vi "STM Reference FGV.vi"(7 "command":enum16{"Set", "Get"}(ring)=enum."Get", 8 "error in":errorcluster, 9 "STM queue in":refnum<queue>, 10 "TCP listener ID in":refnum<k5>, 11 "TCP connection ID in":refnum<k5>) -> (0 "error ou":errorcluster, 1 "STM queue out":refnum<queue>, 2 "TCP listener ID out":refnum<k5>, 3 "TCP connection ID out":refnum<k5>)   [LabVIEW 2017, in "WinHost.lvlib"]
uses:
  WinHost.lvlib
  Private TypeDefs/STM Queue Element.ctl
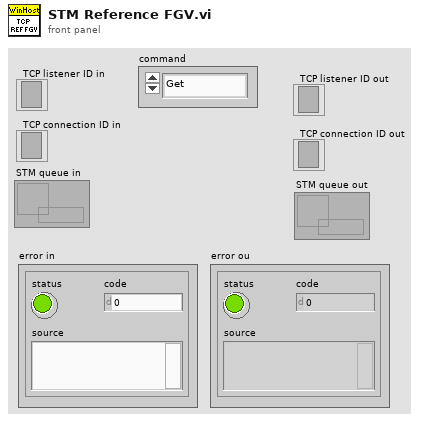
[diagram p1: front panel]
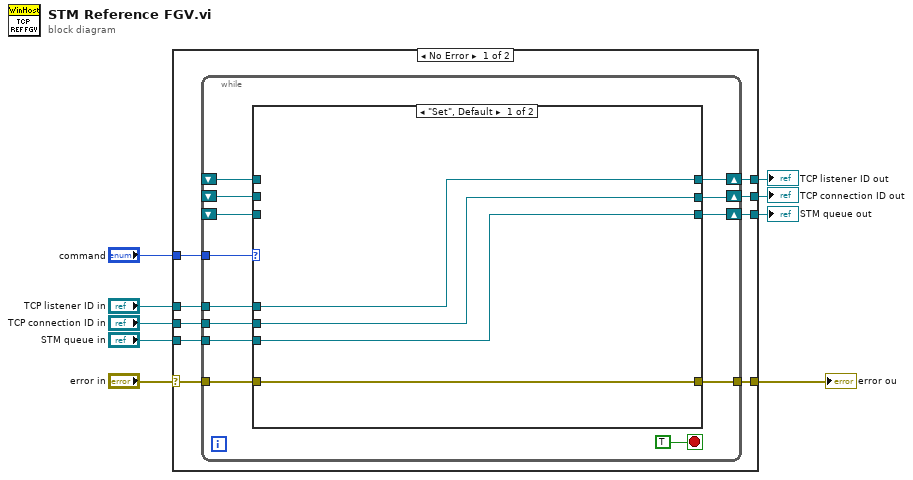
[diagram p0: block diagram]
diagram:
  n1 = case shown="No Error" "error in" {
    selector: "error in" -> [w17 w40]
    tunnel: [w14 w40] -> w8
    tunnel: "command" -> [w18 _]
    tunnel: "TCP listener ID in" -> [w16 _]
    tunnel: "TCP connection ID in" -> [w15 _]
    tunnel: [w13 _] -> w4
    tunnel: [w12 _] -> w3
    tunnel: [w11 _] -> w1
    tunnel: "STM queue in" -> [w10 _]
    frame No Error {
      n2 = while {
        tunnel: w18 -> [w30]
        tunnel: w17 -> [w29]
        tunnel: w16 -> [w28]
        tunnel: w15 -> [w27]
        shift-right: [w25] -> w12
        shift-left: _ -> [w23]
        shift-right: [w26] -> w13
        shift-left: _ -> [w24]
        tunnel: [w22] -> w14
        tunnel: w10 -> [w20]
        shift-right: [w21] -> w11
        shift-left: _ -> [w19]
        stop <- TRUE stop-if-true
        n3 = case shown="\"Set\", Default" w30 {
          tunnel: w29 -> [w33 w37]
          tunnel: w28 -> [w35 _]
          tunnel: w27 -> [w34 _]
          tunnel: [w35 w39] -> w26
          tunnel: [w34 w38] -> w25
          tunnel: w24 -> [_ w39]
          tunnel: w23 -> [_ w38]
          tunnel: [w33 w37] -> w22
          tunnel: [w32 w36] -> w21
          tunnel: w20 -> [w32 _]
          tunnel: w19 -> [_ w36]
          frame "Set", Default {
          }
          frame "Get" {
          }
        }
      }
    }
    frame Error {
    }
  }
  "error ou" <- w8
  "TCP listener ID out" <- w4
  "TCP connection ID out" <- w3
  "STM queue out" <- w1
